vi "Open.vi"(0 "ip":string, 1 "username":string, 2 "password":string, 5 "port":u16, 11 "error in (no error)":errorcluster) -> (4 "handle out":T1, 15 "error out":errorcluster)   [LabVIEW 2018, in "DCAF_JSON_RPC_client.lvlib"]
uses:
  DCAF_JSON_RPC_client.lvlib
  handle.ctl
  <vilib>/httpClient/ClientHandle.ctl
  <vilib>/httpClient/LabVIEWHTTPClient.lvlib
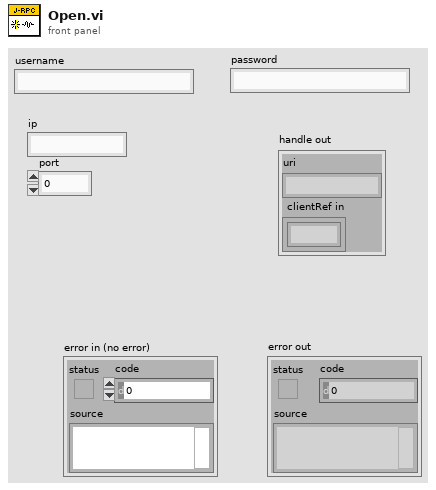
[diagram p1: front panel]
types:
  T1 = typedef "DCAF_JSON_RPC_client.lvlib/handle.ctl" = cluster{"uri":string, " clientRef in":T2}
  T2 = typedef "LabVIEWHTTPClient.lvlib/ClientHandle.ctl" = refnum<k1>
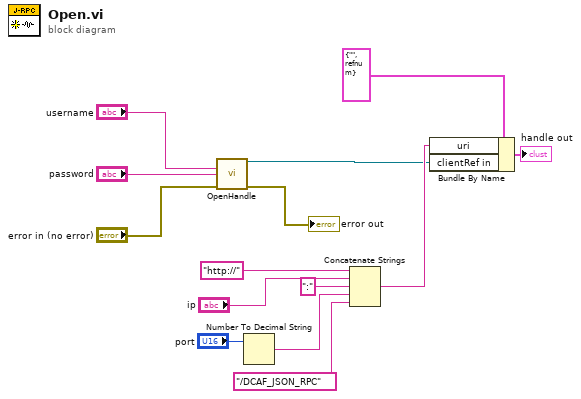
[diagram p0: block diagram]
diagram:
  n1 = call <vilib>:"OpenHandle.vi"("username"="username", "password"="password", "error in (no error)"="error in (no error)") -> ("client handle out"=w3:T2, "error out"=→"error out":errorcluster)  [unwired: 11 in]
  n2 = Number To Decimal String(number="port") -> (decimal integer string=w7:string)  [unwired: 1 in]
  n3 = Concatenate Strings("http://", "ip", ":" ("string"), w7, "/DCAF_JSON_RPC" ("string")) -> (w4:string)
  n4 = Bundle By Name(cluster=T1 {"uri"="", " clientRef in"=refnum} ("handle"), "uri"=w4, "clientRef in"=w3) -> (→"handle out":T1)
